vi "Evaluate Interpolating Polynomial.vi"(9 "xi":dbl[](array[numeric]) format="%_6g", 11 "piecewise polynomial":T1 {"x locations" format="%.4g"; "coefficients" format="%.4g"}) -> (0 "error":i32, 3 "yi":dbl[](array[numeric]) format="%_6g")   [LabVIEW 2010, in "NI_Gmath.lvlib"]
doc: "Takes the <B>piecewise polynomial</B> cluster and computes the interpolated values <B>yi</B> at each <B>xi</B> location."
uses:
  NI_Gmath.lvlib
  in_piecewise interp poly control.ctl
  Scalar Polynomial Evaluation (DBL).vi
  NI_AALPro.lvlib
panel:
  # "Evaluate Interpolating Polynomial"
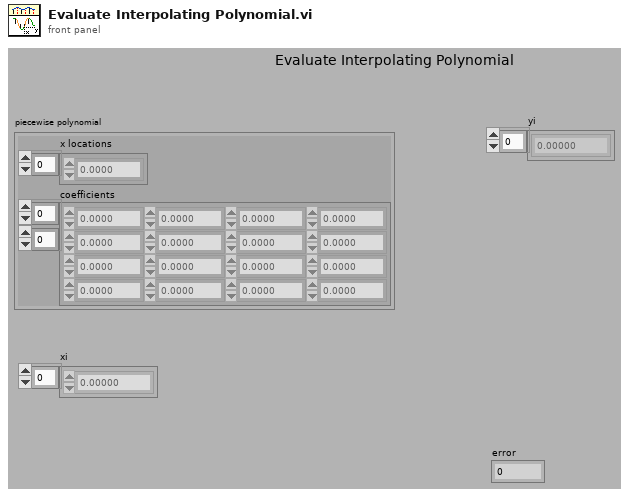
[diagram p1: front panel]
types:
  T1 = typedef "NI_Gmath.lvlib/in_piecewise interp poly control.ctl" = cluster{"x locations":dbl[], "coefficients":dbl[][]}
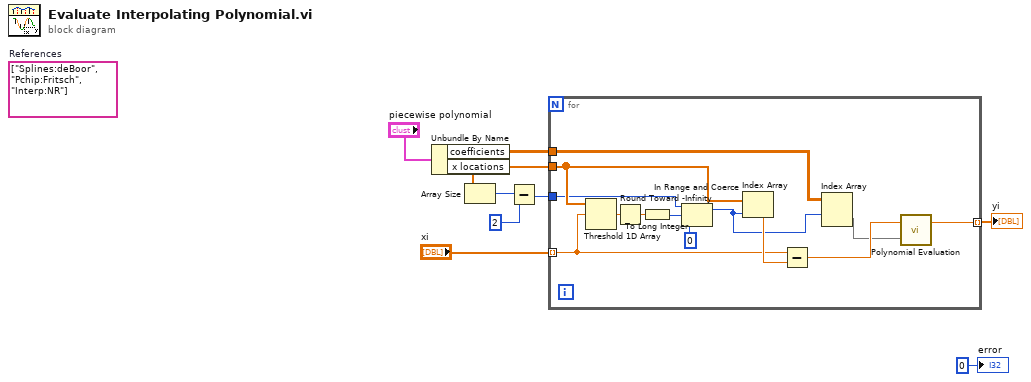
[diagram p0: block diagram]
diagram:
  (unwired) string[] ["Splines:deBoor", "Pchip:Fritsch", "Interp:NR"]  # References
  n1 = Unbundle By Name("piecewise polynomial") -> ("coefficients"=w8:dbl[][], "x locations"=w7:dbl[])
  n2 = Array Size(array=w7) -> (size(s)=w6:i32)
  n3 = Subtract(x=w6, y=2) -> (x-y=w4:i32)
  n4 = for {
    tunnel: w8 -> [w21]
    tunnel: "xi" -> [w14] mode=indexing
    tunnel: w7 -> [w19]
    tunnel: [w17] -> w2 mode=indexing
    tunnel: w4 -> [w11]
    n5 = Threshold 1D Array(2:w14, 3:w19) -> (0:w20:dbl)  [unwired: 1 in]
    n6 = Round Toward -Infinity(1:w20) -> (0:w15:dbl)
    n7 = To Long Integer(number=w15) -> (32bit integer=w13:i32)
    n8 = In Range and Coerce(upper limit=w11, x=w13, lower limit=0) -> (coerced(x)=w12:i32)  [unwired: 1 out]
    n9 = Index Array(array=w19, index=w12) -> (element=w22:dbl)
    n10 = Subtract(x=w14, y=w22) -> (x-y=w18:dbl)
    n11 = Index Array(array=w21, index (row)=w12) -> (element=w16:dbl[])  [unwired: 1 in]
    n12 = call-poly "Polynomial Evaluation.vi"("P(x)"=w16, "a"=w18) -> ("P(a)"=w17:dbl)  [unwired: 1 out]
  }
  "yi" <- w2
  "error" <- 0 ("error")
